vi "Read Starting Buffer Index.vi"(8 "error in":errorcluster, 11 "custom device":T1=18446744073709551615 format="%.0x") -> (0 "error out":errorcluster, 2 "starting buffer index":i32, 3 "custom device out":T1 format="%.0x")   [LabVIEW 2020, in "AIM MIL-STD-1553 Scripting.lvlib"]
doc: "Returns <b>starting buffer index</b>."
uses:
  AIM MIL-STD-1553 Scripting.lvlib
  <vilib>/NI VeriStand/Custom Device API/Custom Device Item Ref.ctl
  Constants.vi
  <vilib>/NI VeriStand/Custom Device API/Custom Device API.lvlib
  <vilib>/NI VeriStand/Custom Device API/Get Item Property (U16).vi
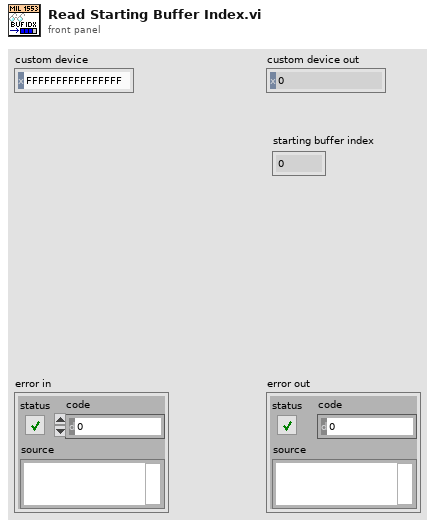
[diagram p1: front panel]
types:
  T1 = typedef "Custom Device API.lvlib/Custom Device Item Ref.ctl" = u64
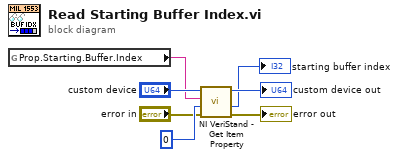
[diagram p0: block diagram]
diagram:
  n1 = global read "Constants.vi" "Prop.Starting.Buffer.Index"() -> (w2:string)
  n2 = call-poly <vilib>:"NI VeriStand - Get Item Property.vi"("error in (no error)"="error in", "Default Value"=i16 0, "Property Name"=w2, "Item Ref in"="custom device") -> ("error out"=→"error out":errorcluster, "Value"=→"starting buffer index":u16, "Item Ref out"=→"custom device out":T1)  [unwired: 4 in, 1 out]
